vi "Init.vi"(8 "error in":errorcluster, 11 "CFG Base in":refnum<class "EL Control Load CFG.lvclass">) -> (0 "error out":errorcluster, 3 "CFG Base out":refnum<class "EL Control Load CFG.lvclass">)   [LabVIEW 2024, in "EL Control Load CFG.lvclass"]
uses:
  EL Control Load CFG.lvclass
  SCPI PE Input.ctl
  EL Control Load CFG.lvclass/EL Control Load CFG.ctl
  <vilib>/Instr/_visa.llb/VISA Configure Serial Port (Instr).vi
  Configurations/CFG Base/CFG Base.lvclass
  D:/git/HAL/HAL/Configurations/CFG Base/CFG Base.lvclass
  D:/git/HAL/HAL/Devices/Eletronic Load 9080/Configurations/Control Load/EL Control Load CFG.lvclass
panel:
  out "Instr Info":variant
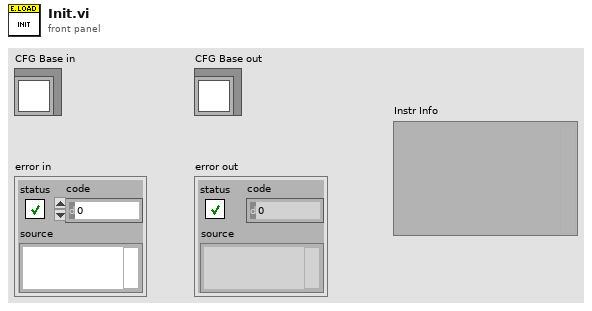
[diagram p1: front panel]
types:
  T1 = typedef "SCPI PE Input.ctl" = cluster{"Action":enum16{"Write", "Query"}, "SCPI":string}
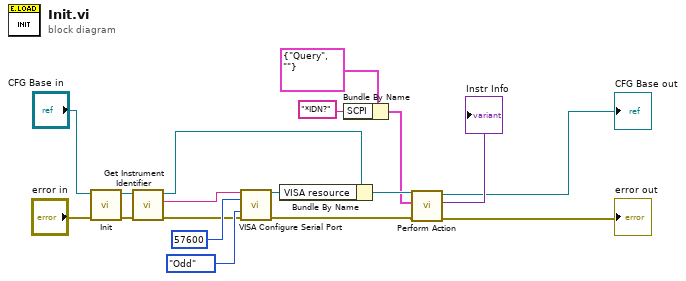
[diagram p0: block diagram]
diagram:
  n1 = call-parent "Init.vi"("error in"="error in", "CFG Base in"="CFG Base in") -> ("error out"=w1:errorcluster, "CFG Base out"=w3:refnum<class "EL Control Load CFG.lvclass">)  [unwired: 8 in]
  n2 = call "Get Instrument Identifier.vi"("CFG Base in"=w3) -> ("Instrument Identifier"=w16:string, "CFG Base out"=w13:refnum<class "EL Control Load CFG.lvclass">)  [unwired: 9 in]
  n3 = call-poly "VISA Configure Serial Port"("VISA resource name"=w16, "baud rate (9600)"=u32 57600, "parity (0:none)"=enum16{"None", "Odd", "Even", "Mark", "Space"}."Odd", "error in (no error)"=w1) -> ("VISA resource name out"=w10:refnum<visa-resource-name>, "error out"=w12:errorcluster)  [unwired: 6 in, 4 out]
  n4 = Bundle By Name(cluster=w13, "VISA resource"=w10) -> (w9:refnum<class "EL Control Load CFG.lvclass">)
  n5 = Bundle By Name(cluster=T1 {"Action"=enum."Query", "SCPI"=""} ("PE Input"), "SCPI"="*IDN?") -> (w6:T1)
  n6 = call-dynamic "Perform Action.vi"("error in"=w12, "Input"=w6, "Control Load CFG in"=w9) -> ("error out"=→"error out":errorcluster, "Output"=→"Instr Info":variant, "Control Load CFG out"=→"CFG Base out":refnum<class "EL Control Load CFG.lvclass">)  [unwired: 6 in]
